vi "TDS RF Power Input Read.vi"(6 "Reference Level (dBm)":dbl, 8 "error in (no error)":errorcluster, 9 "Center Frequency (MHz)":dbl, 10 "Signal InstConfig":string, 11 "Address":string) -> (0 "error out":errorcluster, 3 "Power":dbl)   [LabVIEW 2025, in "Interface Functions.lvlib"]
uses:
  Interface Functions.lvlib
  <instrlib>/Agilent U2000 Series/Agilent U2000 Series.lvlib
panel:
  # "RF Power Input Read"
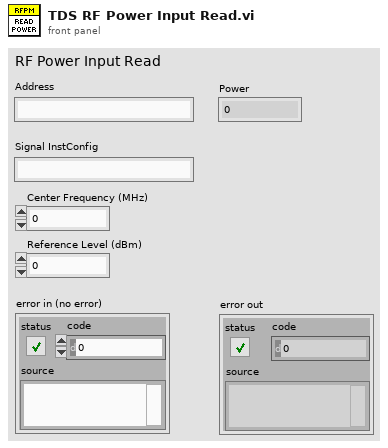
[diagram p1: front panel]
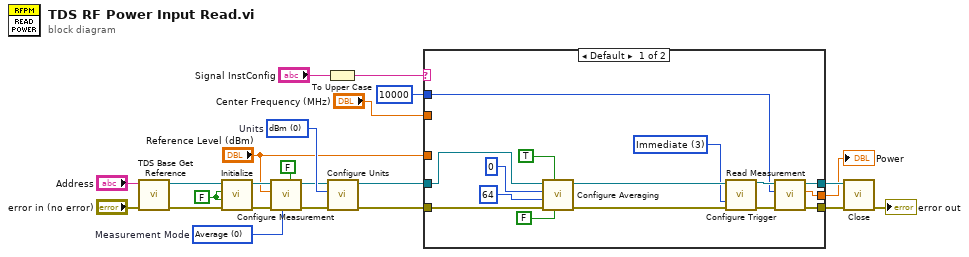
[diagram p0: block diagram]
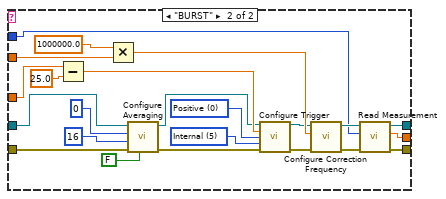
[diagram p2: hidden frame]
diagram:
  w8 = 0 items=["Average", "Normal"]  # Measurement Mode
  w9 = u16 0 items=["dBm", "W"]  # Units
  w12 = FALSE ("ID Query (True)")
  n1 = call "TDS Base Get Reference.vi"("error in (no error)"="error in (no error)", "Address"="Address") -> ("error out"=w15:errorcluster, "Reference"=w13:refnum<visa-resource-name>)  [unwired: 8 in]
  n2 = call <instrlib>:"Initialize.vi"("error in (no error)"=w15, "Reset (True)"=w12, "ID Query (True)"=w12, "VISA resource name"=w13) -> ("error out"=w6:errorcluster, "VISA resource name out"=w7:refnum<visa-resource-name>)  [unwired: 6 in]
  n3 = call <instrlib>:"Configure Measurement.vi"("Enable Gate Feed (T: Enable)"=FALSE, "Measurement Function (0: Average)"=w8, "error in (no error)"=w6, "Expected Value (0)"="Reference Level (dBm)", "VISA resource name"=w7) -> ("error out"=w10:errorcluster, "VISA resource name out"=w5:refnum<visa-resource-name>)  [unwired: 5 in]
  n4 = To Upper Case(1:"Signal InstConfig") -> (0:w20:string)
  n5 = call <instrlib>:"Configure Units.vi"("error in (no error)"=w10, "Units (0: dBm)"=w9, "VISA resource name"=w5) -> ("error out"=w4:errorcluster, "VISA resource name out"=w3:refnum<visa-resource-name>)  [unwired: 1 in, 6 out]
  n6 = case shown="Default" w20 {
    tunnel: [w28 w46] -> w18
    tunnel: [w29 w45] -> w17
    tunnel: [w27 w44] -> w16
    tunnel: w4 -> [w25 w43]
    tunnel: "Reference Level (dBm)" -> [_ w42]
    tunnel: "Center Frequency (MHz)" -> [_ w41]
    tunnel: w3 -> [w26 w40]
    tunnel: u32 10000 ("Timeout (10000 ms)") -> [w30 w39]
    frame Default {
      w31 = 3 items=["Bus", "External", "Hold", "Immediate", "Internal A", "Internal"] ("Trigger Source (3: Immediate)")
      n7 = call <instrlib>:"Configure Averaging.vi"("Auto Averaging (T: Enable)"=FALSE, "Enable Averaging (T: Enable)"=TRUE, "error in (no error)"=w25, "Averaging Count (4)"=64, "Averaging Buffer Size (1)"=0, "VISA resource name"=w26) -> ("error out"=w35:errorcluster, "VISA resource name out"=w34:refnum<visa-resource-name>)  [unwired: 4 in]
      n8 = call <instrlib>:"Configure Trigger.vi"("VISA resource name"=w34, "Trigger Source (3: Immediate)"=w31, "error in (no error)"=w35) -> ("VISA resource name out"=w33:refnum<visa-resource-name>, "error out"=w32:errorcluster)  [unwired: 11 in]
      n9 = call <instrlib>:"Read Measurement.vi"("error in (no error)"=w32, "Timeout (10000 ms)"=w30, "VISA resource name"=w33) -> ("error out"=w28:errorcluster, "Measurement"=w27:dbl, "VISA resource name out"=w29:refnum<visa-resource-name>)  [unwired: 6 in]
    }
    frame "BURST" {
      w57 = 5 items=["Bus", "External", "Hold", "Immediate", "Internal A", "Internal"] ("Trigger Source (3: Immediate)")
      w58 = u16 0 items=["Positive", "Negative"] ("Trigger Slope (0: Positive)")
      n10 = Subtract(x=w42, y=25.0) -> (x-y=w55:dbl)
      n11 = Multiply(x=1000000.0, y=w41) -> (x*y=w53:dbl)
      n12 = call <instrlib>:"Configure Averaging.vi"("Auto Averaging (T: Enable)"=FALSE, "error in (no error)"=w43, "Averaging Count (4)"=16, "Averaging Buffer Size (1)"=0, "VISA resource name"=w40) -> ("error out"=w48:errorcluster, "VISA resource name out"=w47:refnum<visa-resource-name>)  [unwired: 5 in]
      n13 = call <instrlib>:"Configure Trigger.vi"("VISA resource name"=w47, "Trigger Level (0 dBm)"=w55, "Trigger Slope (0: Positive)"=w58, "Trigger Source (3: Immediate)"=w57, "error in (no error)"=w48) -> ("VISA resource name out"=w51:refnum<visa-resource-name>, "error out"=w52:errorcluster)  [unwired: 9 in]
      n14 = call <instrlib>:"Configure Correction Frequency.vi"("error in (no error)"=w52, "Frequency (5E+7 Hz)"=w53, "VISA resource name"=w51) -> ("error out"=w49:errorcluster, "VISA resource name out"=w50:refnum<visa-resource-name>)  [unwired: 7 in]
      n15 = call <instrlib>:"Read Measurement.vi"("error in (no error)"=w49, "Timeout (10000 ms)"=w39, "VISA resource name"=w50) -> ("error out"=w46:errorcluster, "Measurement"=w44:dbl, "VISA resource name out"=w45:refnum<visa-resource-name>)  [unwired: 6 in]
    }
  }
  "Power" <- w16
  n16 = call <instrlib>:"Close.vi"("error in (no error)"=w18, "VISA resource name"=w17) -> ("error out"=→"error out":errorcluster)  [unwired: 9 in]
